vi "[Global] ExtractedAnalizedImage.vi"() -> ()   [LabVIEW 2019]
panel:
  out "ExtractedAnalizedImageArray":string[](array[string])=["ExtractedAnalizedImage0", "ExtractedAnalizedImage1", "ExtractedAnalizedImage2", "ExtractedAnalizedImage3", "ExtractedAnalizedImage4", "ExtractedAnalizedImage5", "ExtractedAnalizedImage6", "ExtractedAnalizedImage7"]
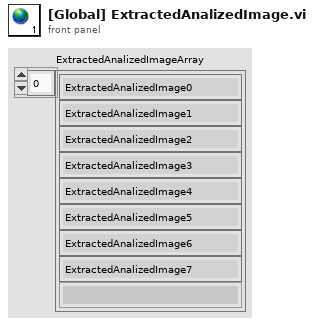
[diagram p1: front panel]
diagram:
